vi "PID.vi"(7 "PID Gains":cluster{"P":dbl, "I":dbl, "D":dbl}, 9 "Reset I":bool, 10 "dt":dbl, 11 "Error":dbl) -> (3 "result":dbl)   [LabVIEW 2017]
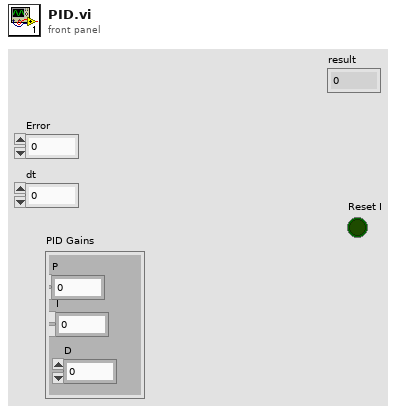
[diagram p1: front panel]
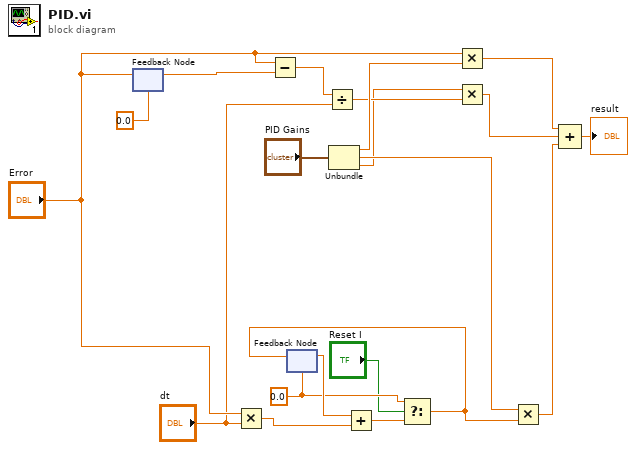
[diagram p0: block diagram]
diagram:
  w2 = 0.0
  n1 = feedback #1(0.0) -> (w18:dbl)
  n2 = feedback-in #1("Error") -> ()
  n3 = Multiply(x="Error", y="dt") -> (x*y=w15:dbl)
  n4 = Subtract(x="Error", y=w18) -> (x-y=w12:dbl)
  n5 = feedback #2(w2) -> (w17:dbl)
  n6 = Divide(x=w12, y="dt") -> (x/y=w11:dbl)
  n7 = Unbundle("PID Gains") -> ("P"=w19:dbl, "I"=w14:dbl, "D"=w10:dbl)
  n8 = Add(x=w17, y=w15) -> (x+y=w3:dbl)
  n9 = Select(t=w2, s="Reset I", f=w3) -> (s? t:f=w4:dbl)
  n10 = feedback-in #2(w4) -> ()
  n11 = Multiply(x="Error", y=w19) -> (x*y=w9:dbl)
  n12 = Multiply(x=w10, y=w11) -> (x*y=w8:dbl)
  n13 = Multiply(x=w14, y=w4) -> (x*y=w7:dbl)
  n14 = Compound Arithmetic op=ADD(w9, w8, w7) -> (→"result":dbl)
